vi "Write Plot Name.vi"(4 "error in (no error)":errorcluster, 5 "Value":string[](array[string]), 6 "Container State":T2, 7 "Display State In":T1) -> (0 "error out":errorcluster, 3 "Display State Out":T1)   [LabVIEW 2013, in "Configurable Buffer.xctl"]
uses:
  Configurable Buffer.xctl
  <vilib>/_xctls/Container State.ctl
  State.ctl
  <vilib>/_xctls/XControlSupport.lvlib
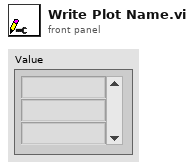
[diagram p1: front panel]
types:
  T1 = typedef "Configurable Buffer.xctl/State.ctl" = cluster{"Plot Ref":refnum<vi>, "History":i32}
  T2 = typedef "XControlSupport.lvlib/Container State.ctl" = cluster{"Indicator?":bool, "Run Mode?":bool, " Refnum":refnum<vi>}
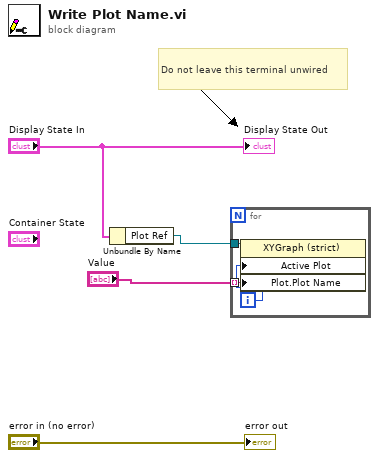
[diagram p0: block diagram]
diagram:
  # "Do not leave this terminal unwired"
  n1 = Unbundle By Name("Display State In") -> ("Plot Ref"=w2:refnum<vi>)
  n2 = for {
    tunnel: w2 -> [w7]
    tunnel: "Value" -> [w5] mode=indexing
    i -> [w6]
    n3 = property class="XYGraph (strict)"(reference=w7, "Active Plot"=w6, "Plot.Plot Name"=w5) -> ()  [unwired: 1 in, 2 out]
  }
  "error out" <- "error in (no error)"
  "Display State Out" <- "Display State In"
